vi "Tidal Eng-Modbus Data.vi"(8 "error in (no error)":errorcluster, 10 "IP Address":string, 11 "Modbus master in":refnum<class "Modbus Master.lvclass">) -> (0 "error out":errorcluster, 1 "Tenney Data":string[][](array[string]), 2 "Tenney Environmental Chamber Data Output":T1, 3 "Modbus master out":refnum<class "Modbus Master.lvclass">)   [LabVIEW 2023]
uses:
  Type Definitions/Tenney Modbus Registers.ctl
  <vilib>/NI/Modbus Library/API/Master/Modbus Master.lvclass
  Type Definitions/Tenney Environmental Chamber Data.ctl
panel:
  in  "Chamber ON/OFF":T2=40600 items=["Ch1 Setpoint"=40100, "Ch1 Process Variable"=40103, "Ch2 Setpoint"=40200, "Ch2 Process Variable"=40203, "Ch3 Setpoint"=40300, "Ch3 Process Variable"=40303, "All Events Mask"=40500, "Run State"=40600]
  in  "Frequency Process Variable":T2=40303 items=["Ch1 Setpoint"=40100, "Ch1 Process Variable"=40103, "Ch2 Setpoint"=40200, "Ch2 Process Variable"=40203, "Ch3 Setpoint"=40300, "Ch3 Process Variable"=40303, "All Events Mask"=40500, "Run State"=40600]
  in  "Frequency Setpoint":T2=40300 items=["Ch1 Setpoint"=40100, "Ch1 Process Variable"=40103, "Ch2 Setpoint"=40200, "Ch2 Process Variable"=40203, "Ch3 Setpoint"=40300, "Ch3 Process Variable"=40303, "All Events Mask"=40500, "Run State"=40600]
  in  "Humidity Process Variable":T2=40203 items=["Ch1 Setpoint"=40100, "Ch1 Process Variable"=40103, "Ch2 Setpoint"=40200, "Ch2 Process Variable"=40203, "Ch3 Setpoint"=40300, "Ch3 Process Variable"=40303, "All Events Mask"=40500, "Run State"=40600]
  in  "Humidity Setpoint":T2=40200 items=["Ch1 Setpoint"=40100, "Ch1 Process Variable"=40103, "Ch2 Setpoint"=40200, "Ch2 Process Variable"=40203, "Ch3 Setpoint"=40300, "Ch3 Process Variable"=40303, "All Events Mask"=40500, "Run State"=40600]
  in  "Temperature Process Variable":T2=40103 items=["Ch1 Setpoint"=40100, "Ch1 Process Variable"=40103, "Ch2 Setpoint"=40200, "Ch2 Process Variable"=40203, "Ch3 Setpoint"=40300, "Ch3 Process Variable"=40303, "All Events Mask"=40500, "Run State"=40600]
  in  "Temperature Setpoint":T2=40100 items=["Ch1 Setpoint"=40100, "Ch1 Process Variable"=40103, "Ch2 Setpoint"=40200, "Ch2 Process Variable"=40203, "Ch3 Setpoint"=40300, "Ch3 Process Variable"=40303, "All Events Mask"=40500, "Run State"=40600]
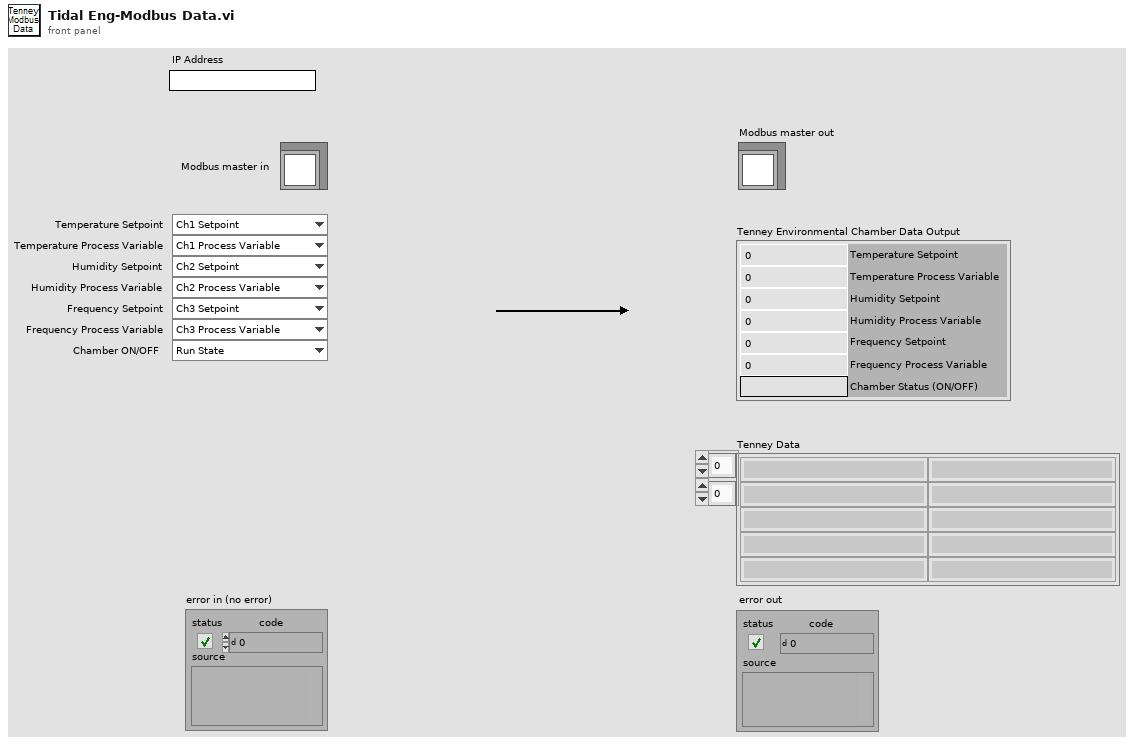
[diagram p1: front panel]
types:
  T1 = typedef "Tenney Environmental Chamber Data.ctl" = cluster{"Temperature Setpoint":dbl, "Temperature Process Variable":dbl, "Humidity Setpoint":dbl, "Humidity Process Variable":dbl, "Frequency Setpoint":dbl, "Frequency Process Variable":dbl, "Chamber Status (ON/OFF)":string}
  T2 = typedef "Tenney Modbus Registers.ctl" = u16
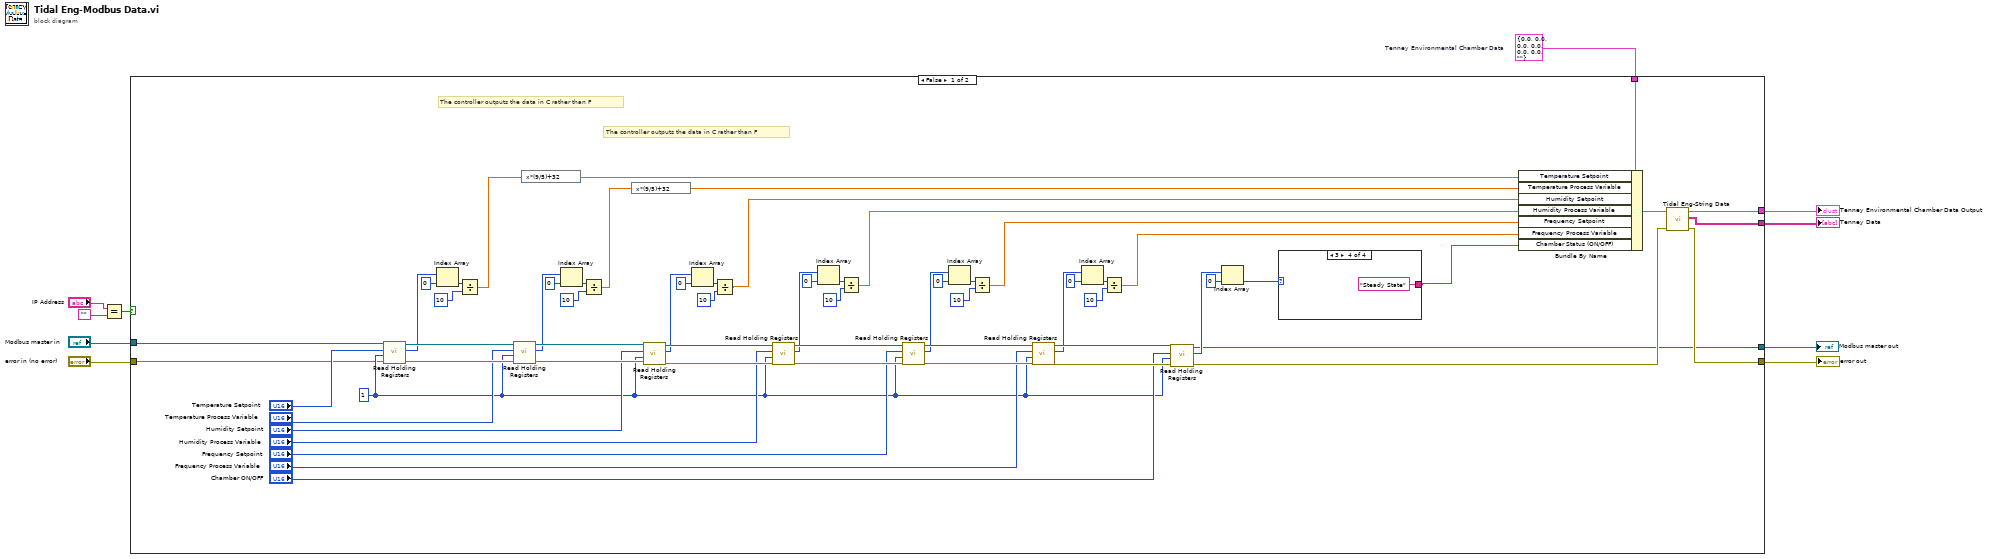
[diagram p0: block diagram]
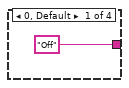
[diagram p2: hidden frame]
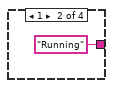
[diagram p3: hidden frame]
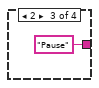
[diagram p4: hidden frame]
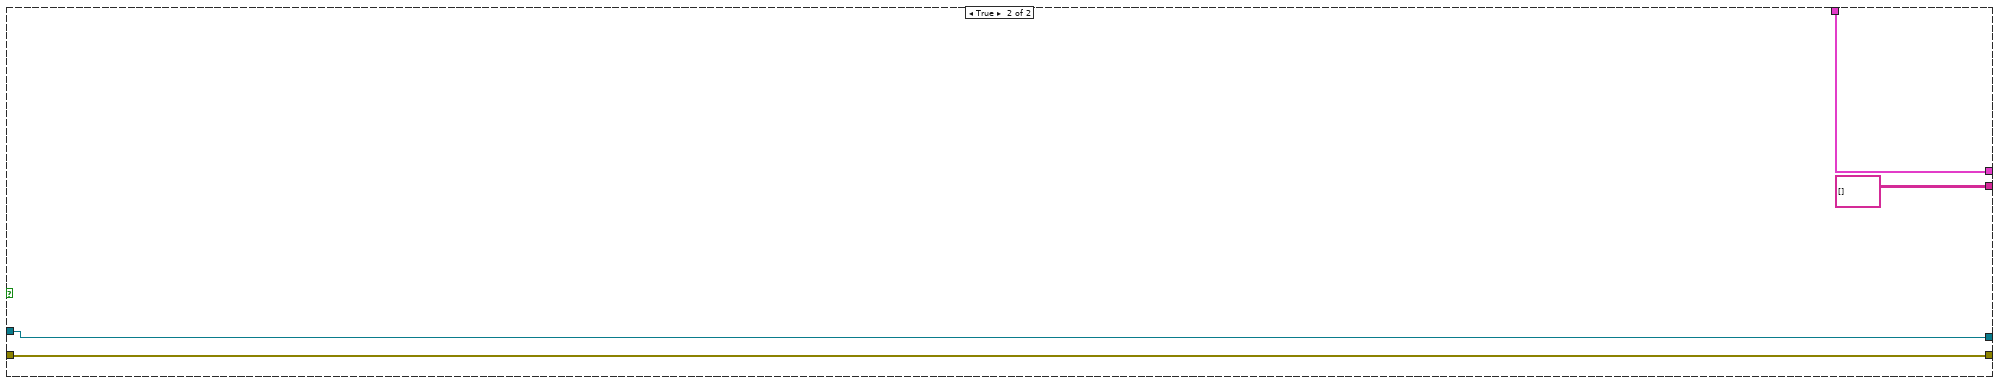
[diagram p5: hidden frame]
diagram:
  w1 = T1 {"Temperature Setpoint"=0.0, "Temperature Process Variable"=0.0, "Humidity Setpoint"=0.0, "Humidity Process Variable"=0.0, "Frequency Setpoint"=0.0, "Frequency Process Variable"=0.0, "Chamber Status (ON/OFF)"=""}  # Tenney Environmental Chamber Data
  n1 = Equal?(x="IP Address", y="") -> (x = y?=w5:bool)
  n2 = case shown="False" w5 {
    tunnel: [w18 w80] -> w10
    tunnel: [w17 string[][] [] ("Tenney Data")] -> w9
    tunnel: [w15 w83] -> w8
    tunnel: [w14 w82] -> w4
    tunnel: "error in (no error)" -> [w13 w83]
    tunnel: "Modbus master in" -> [w12 w82]
    tunnel: w1 -> [w11 w80]
    frame False {
      w20 = u16 1 ("number of inputs")
      # "The controller outputs the data in C rather than F"
      # "The controller outputs the data in C rather than F"
      n3 = call-dynamic "Read Holding Registers.vi"("error in"=w13, "number of inputs"=w20, "starting address"="Temperature Setpoint", "Modbus master in"=w12) -> ("error out"=w69:errorcluster, "register values"=w56:u16[], "Modbus master out"=w74:refnum<class "Modbus Master.lvclass">)  [unwired: 5 in]
      n4 = Index Array(array=w56, index=0) -> (element=w54:u16)
      n5 = Divide(x=w54, y=u16 10) -> (x/y=w26:dbl)
      n6 = call-dynamic "Read Holding Registers.vi"("error in"=w69, "number of inputs"=w20, "starting address"="Temperature Process Variable", "Modbus master in"=w74) -> ("error out"=w68:errorcluster, "register values"=w51:u16[], "Modbus master out"=w73:refnum<class "Modbus Master.lvclass">)  [unwired: 5 in]
      n7 = expression code="x*(9/5)+32"(w26) -> (w25:dbl)
      n8 = Index Array(array=w51, index=0) -> (element=w53:u16)
      n9 = Divide(x=w53, y=u16 10) -> (x/y=w24:dbl)
      n10 = expression code="x*(9/5)+32"(w24) -> (w23:dbl)
      n11 = call-dynamic "Read Holding Registers.vi"("error in"=w68, "number of inputs"=w20, "starting address"="Humidity Setpoint", "Modbus master in"=w73) -> ("error out"=w67:errorcluster, "register values"=w48:u16[], "Modbus master out"=w72:refnum<class "Modbus Master.lvclass">)  [unwired: 5 in]
      n12 = Index Array(array=w48, index=0) -> (element=w49:u16)
      n13 = Divide(x=w49, y=u16 10) -> (x/y=w30:dbl)
      n14 = call-dynamic "Read Holding Registers.vi"("error in"=w67, "number of inputs"=w20, "starting address"="Humidity Process Variable", "Modbus master in"=w72) -> ("error out"=w66:errorcluster, "register values"=w45:u16[], "Modbus master out"=w71:refnum<class "Modbus Master.lvclass">)  [unwired: 5 in]
      n15 = Index Array(array=w45, index=0) -> (element=w47:u16)
      n16 = Divide(x=w47, y=u16 10) -> (x/y=w29:dbl)
      n17 = call-dynamic "Read Holding Registers.vi"("error in"=w66, "number of inputs"=w20, "starting address"="Frequency Setpoint", "Modbus master in"=w71) -> ("error out"=w65:errorcluster, "register values"=w42:u16[], "Modbus master out"=w70:refnum<class "Modbus Master.lvclass">)  [unwired: 5 in]
      n18 = Index Array(array=w42, index=0) -> (element=w43:u16)
      n19 = Divide(x=w43, y=u16 10) -> (x/y=w28:dbl)
      n20 = call-dynamic "Read Holding Registers.vi"("error in"=w65, "number of inputs"=w20, "starting address"="Frequency Process Variable", "Modbus master in"=w70) -> ("error out"=w58:errorcluster, "register values"=w39:u16[], "Modbus master out"=w59:refnum<class "Modbus Master.lvclass">)  [unwired: 5 in]
      n21 = Index Array(array=w39, index=0) -> (element=w41:u16)
      n22 = Divide(x=w41, y=u16 10) -> (x/y=w27:dbl)
      n23 = call-dynamic "Read Holding Registers.vi"("error in"=w58, "number of inputs"=w20, "starting address"="Chamber ON/OFF", "Modbus master in"=w59) -> ("error out"=w16:errorcluster, "register values"=w37:u16[], "Modbus master out"=w14:refnum<class "Modbus Master.lvclass">)  [unwired: 5 in]
      n24 = Index Array(array=w37, index=0) -> (element=w22:u16)
      n25 = case shown="3" w22 {
        tunnel: ["Off" "Running" "Pause" "Steady State"] -> w21
        frame 0, Default {
        }
        frame 1 {
        }
        frame 2 {
        }
        frame 3 {
        }
      }
      n26 = Bundle By Name(cluster=w11, "Temperature Setpoint"=w25, "Temperature Process Variable"=w23, "Humidity Setpoint"=w30, "Humidity Process Variable"=w29, "Frequency Setpoint"=w28, "Frequency Process Variable"=w27, "Chamber Status (ON/OFF)"=w21) -> (w19:T1)
      n27 = call "Tidal Eng-String Data.vi"("error in (no error)"=w16, "Tenney Environmental Chamber Data Input"=w19) -> ("error out"=w15:errorcluster, "Tenney Data"=w17:string[][], "Tenney Environmental Chamber Data Output"=w18:T1)  [unwired: 7 in]
    }
    frame True {
    }
  }
  "error out" <- w8
  "Tenney Environmental Chamber Data Output" <- w10
  "Tenney Data" <- w9
  "Modbus master out" <- w4
